vi "sub_done_fgv.vi"(7 "cmd":enum16{"ini", "write", "read"}(ring), 8 "error in":errorcluster, 10 "off_track":bool, 11 "input":bool) -> (0 "error out":errorcluster, 1 "range_val":i32, 2 "done_val":i32)   [LabVIEW 2018]
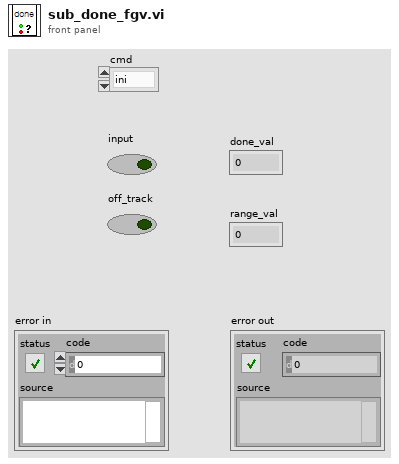
[diagram p1: front panel]
types:
  T1 = typedef "ctr-ref.ctl" = cluster{"connected":refnum<vi>, "start":refnum<vi>, "read_data":refnum<vi>, "Target":refnum<vi>, "play_type":refnum<vi>, "dt_daq":refnum<vi>, "dt_tcp":refnum<vi>, "timer":refnum<vi>, "States":refnum<vi>, "angle_limit":refnum<vi>, "Initial States":refnum<vi>}
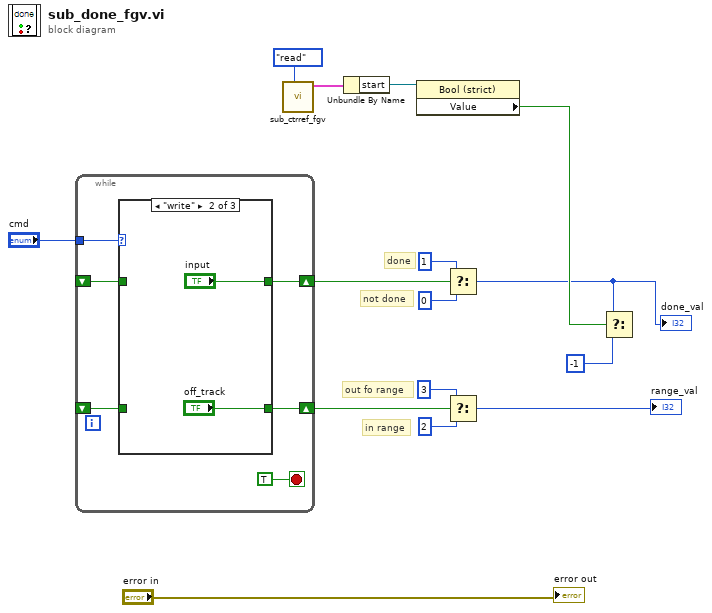
[diagram p0: block diagram]
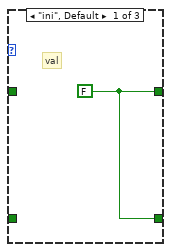
[diagram p2: hidden frame]
diagram:
  # "out fo range"
  # "in range"
  # "not done"
  # "done"
  n1 = while {
    tunnel: "cmd" -> [w20]
    shift-right: [w19] -> w5
    shift-left: _ -> [w18]
    shift-right: [w17] -> w7
    shift-left: _ -> [w16]
    stop <- TRUE stop-if-true
    n2 = case shown="\"write\"" w20 {
      tunnel: [w22 "input" w26] -> w19
      tunnel: w18 -> [_ _ w26]
      tunnel: [w22 "off_track" w25] -> w17
      tunnel: w16 -> [_ _ w25]
      frame "ini", Default {
        w22 = FALSE
        # "val"
      }
      frame "write" {
      }
      frame "read" {
      }
    }
  }
  n3 = call "sub_ctrref_fgv.vi"("cmd"=enum16{"write", "read"}."read") -> ("ctr_out"=w13:T1)  [unwired: 10 in]
  n4 = Unbundle By Name(w13) -> ("start"=w12:refnum<vi>)
  n5 = property class="Bool (strict)"(reference=w12) -> ("Value"=w11:bool)  [unwired: 1 in, 2 out]
  n6 = Select(t=1, s=w5, f=0) -> (s? t:f=w1:i32)
  "done_val" <- w1
  n7 = Select(t=3, s=w7, f=2) -> (s? t:f=→"range_val":i32)
  n8 = Select(t=w1, s=w11, f=-1) -> ()  [unwired: 1 out]
  "error out" <- "error in"
